vi "simulatorControlEncodeErForce.vi"(5 "degubBall":bool=TRUE, 6 "replaceRobots":bool, 8 "error in (no error)":errorcluster, 9 "Ball":refnum<class "Ball.lvclass">, 10 "grSIM replacement":T1, 11 "Communication in":refnum<class "Communication.lvclass">) -> (0 "error out":errorcluster, 2 "SimulatorControlArray":u8[](array[numeric]), 3 "Communication out":refnum<class "Communication.lvclass">)   [LabVIEW 2023, in "Communication.lvclass"]
uses:
  Communication.lvclass
  Controls/grSimReplacement.ctl
  grSim Packet Command UDP Test Folder/grSim/grSim RobotReplacement.ctl
  grSim Packet Command UDP Test Folder/grSim/grSim_BallReplacement.ctl
  Ball_class/Ball.lvclass
  C:/Users/ebert/Documents/codes/SSL/repo/SSL_AI/Object_class/Object.lvclass
  Object_class/Object.lvclass/Object.ctl
  Object_class/Read x.vi
  Object_class/Read y.vi
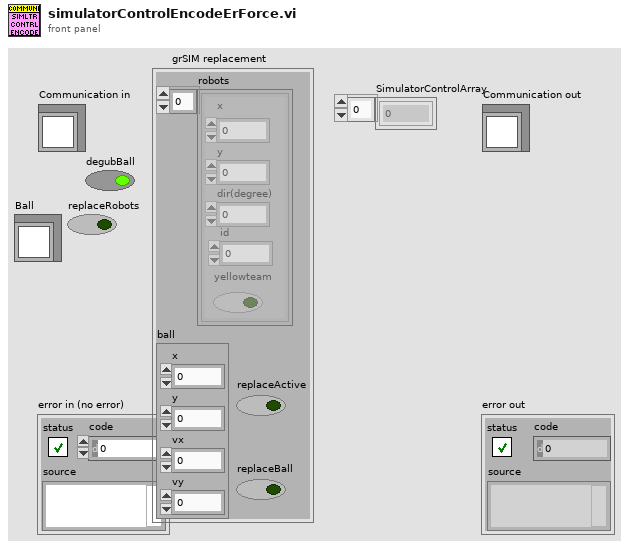
[diagram p1: front panel]
types:
  T1 = typedef "grSimReplacement.ctl" = cluster{"robots":T2[], "ball":T3, "replaceBall":bool, "replaceActive":bool}
  T2 = typedef "grSim RobotReplacement.ctl" = cluster{"x":dbl, "y":dbl, "dir(degree)":dbl, "yellowteam":bool, "id":u32}
  T3 = typedef "grSim_BallReplacement.ctl" = cluster{"x":dbl, "y":dbl, "vx":dbl, "vy":dbl}
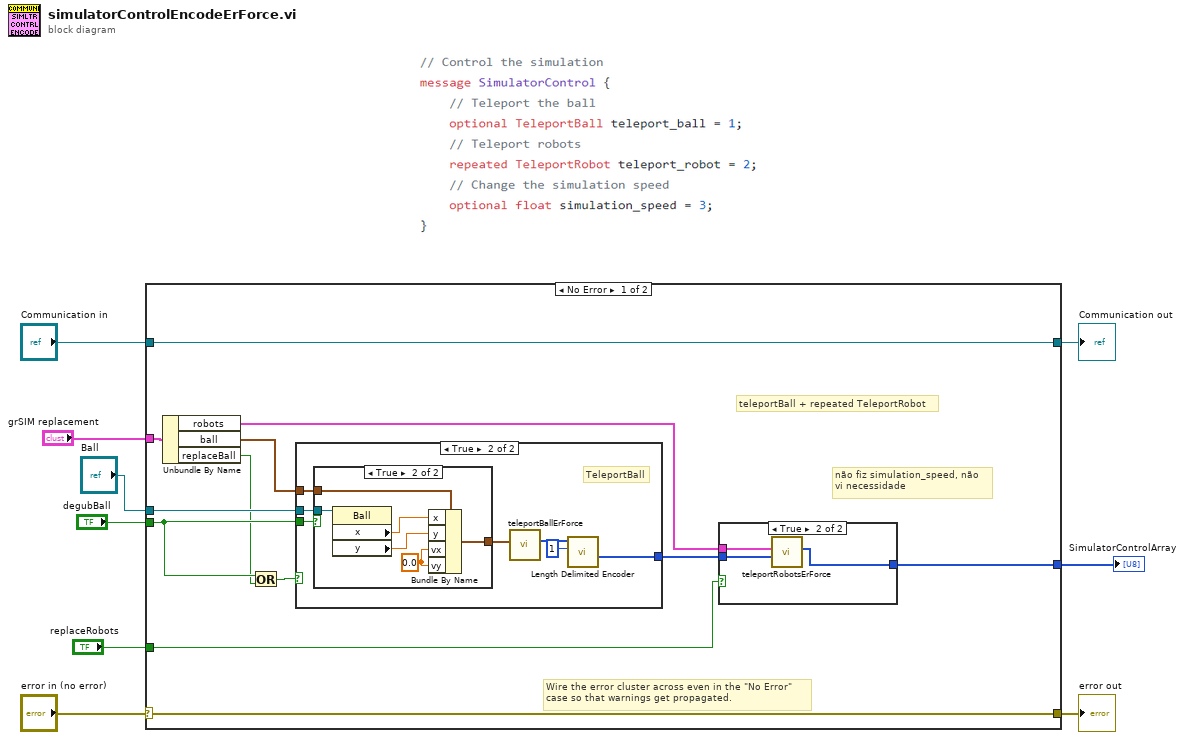
[diagram p0: block diagram]
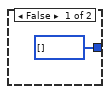
[diagram p3: hidden frame]
diagram:
  n1 = case shown="No Error" "error in (no error)" {
    selector: "error in (no error)" -> [w20 w42]
    tunnel: [w20 w42] -> w8
    tunnel: [w21 w41] -> w6
    tunnel: "Communication in" -> [w21 w41]
    tunnel: "grSIM replacement" -> [w16 _]
    tunnel: [w15 _] -> w4
    tunnel: "degubBall" -> [w13 _]
    tunnel: "Ball" -> [w12 _]
    tunnel: "replaceRobots" -> [w11 _]
    frame No Error {
      # "não fiz simulation_speed, não\nvi necessidade"
      # "teleportBall + repeated TeleportRobot"
      # "Wire the error cluster across even in the \"No Error\"\ncase so that warnings get propagated."
      n2 = Unbundle By Name(w16) -> ("robots"=w18:T2[], "ball"=w17:T3, "replaceBall"=w10:bool)
      n3 = Or(x=w13, y=w10) -> (x .or. y?=w14:bool)
      n4 = case shown="True" w14 {
        tunnel: [u8[] [] ("Array") w31] -> w19
        tunnel: w17 -> [_ w29]
        tunnel: w13 -> [_ w30]
        tunnel: w12 -> [_ w28]
        frame False {
        }
        frame True {
          # "TeleportBall"
          n5 = case shown="True" w30 {
            tunnel: w29 -> [w34 w40]
            tunnel: w28 -> [_ w39]
            tunnel: [w34 w35] -> w27
            frame False {
            }
            frame True {
              w36 = 0.0 ("vx")
              n6 = property class="Ball"(reference=w39) -> ("x"=w38:dbl, "y"=w37:dbl)  [unwired: 1 in, 2 out]
              n7 = Bundle By Name(cluster=w40, "x"=w38, "y"=w37, "vx"=w36, "vy"=w36) -> (w35:T3)
            }
          }
          n8 = call "teleportBallErForce.vi"("ballReplacement"=w27) -> ("teleportBallArray"=w33:u8[])  [unwired: 8 in, 2 out]
          n9 = call "Length Delimited Encoder.vi"("Key"=u32 1, "Array In to be added"=w33) -> ("Array"=w31:u8[])  [unwired: 9 in]
        }
      }
      n10 = case shown="True" w11 {
        tunnel: w19 -> [w22 w25]
        tunnel: w18 -> [_ w24]
        tunnel: [w22 w23] -> w15
        frame False {
        }
        frame True {
          n11 = call "teleportRobotsErForce.vi"("Original Array In"=w25, "robots"=w24) -> ("teleportedRobotsArray"=w23:u8[])  [unwired: 7 in, 2 out]
        }
      }
    }
    frame Error {
    }
  }
  "error out" <- w8
  "Communication out" <- w6
  "SimulatorControlArray" <- w4
